vi "detector_de_umbral.vi"() -> ()   [LabVIEW 2016]
uses:
  <vilib>/Analysis/2dsp.llb/1D Cross Correlation (DBL).vi
  <vilib>/Analysis/NI_AALPro.lvlib
panel:
  out "y(n)":i16
  out "Waveform Chart":dbl(graph)
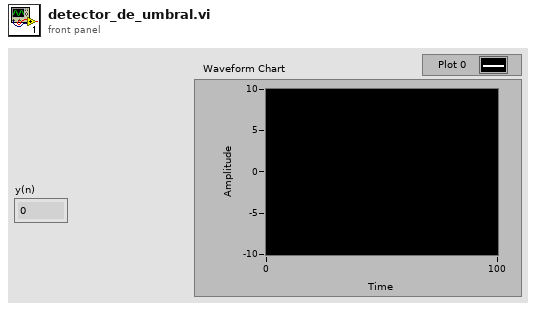
[diagram p1: front panel]
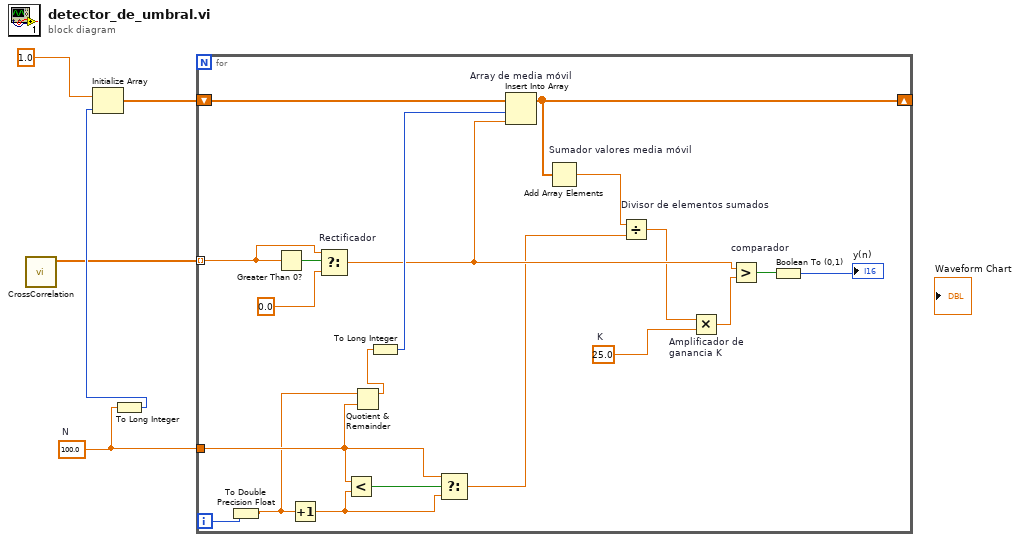
[diagram p0: block diagram]
diagram:
  w3 = 100.0  # N
  n1 = call-poly <vilib>:"CrossCorrelation.vi"() -> ("Rxy"=w1:dbl[])  [unwired: 10 in, 1 out]
  n2 = To Long Integer(number=w3) -> (32bit integer=w2:i32)
  n3 = Initialize Array(1.0, w2) -> (w4:dbl[])
  n4 = for {
    shift-right: [w17] -> _
    shift-left: w4 -> [w25]
    tunnel: w3 -> [w22]
    tunnel: w1 -> [w8] mode=indexing
    i -> [w24]
    w7 = 25.0  # K
    n5 = To Double Precision Float(number=w24) -> (double precision float=w20:dbl)
    n6 = Greater Than 0?(x=w8) -> (x > 0?=w11:bool)
    n7 = Increment(x=w20) -> (x+1=w21:dbl)
    n8 = Select "Rectificador"(t=w8, s=w11, f=0.0) -> (s? t:f=w15:dbl)
    n9 = Less?(x=w22, y=w21) -> (x < y?=w23:bool)
    n10 = Quotient & Remainder(x=w20, y=w22) -> (x-y*floor(x/y)=w19:dbl)  [unwired: 1 out]
    n11 = To Long Integer(number=w19) -> (32bit integer=w18:i32)
    n12 = Select(t=w22, s=w23, f=w21) -> (s? t:f=w13:dbl)
    n13 = Insert Into Array "Array de media móvil"(array=w25, index=w18, new element=w15) -> (w17:dbl[])
    n14 = Add Array Elements "Sumador valores media móvil"(numeric array=w17) -> (sum=w6:dbl)
    n15 = Divide "Divisor de elementos sumados"(x=w6, y=w13) -> (x/y=w14:dbl)
    n16 = Multiply "Amplificador de ganancia K"(x=w14, y=w7) -> (x*y=w16:dbl)
    n17 = Greater? "comparador"(x=w15, y=w16) -> (0:w10:bool)
    n18 = Boolean To (0,1)(Boolean=w10) -> (0, 1=→"y(n)":i16)
  }
